vi "TC10 Update.vi"(5 "TC10 State LED ref":refnum<vi>, 7 "INTERFACE NAME ref":refnum<vi>, 8 "error in":errorcluster, 11 "XNET Session in":refnum<k21>) -> (0 "error out":errorcluster, 3 "XNET Session out":refnum<k21>)   [LabVIEW 2025, in "Automotive Ethernet Bus Monitor UI.lvlib"]
doc: "Update the TC10 session and state LED."
uses:
  Automotive Ethernet Bus Monitor UI.lvlib
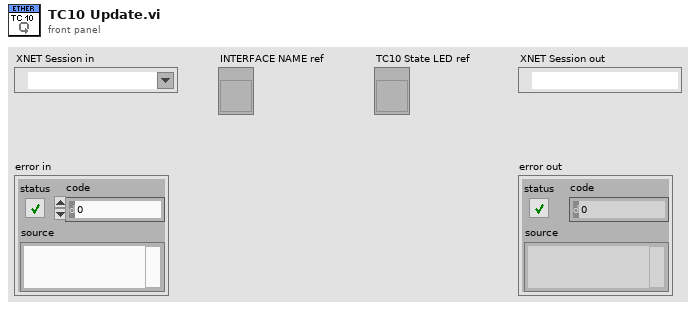
[diagram p1: front panel]
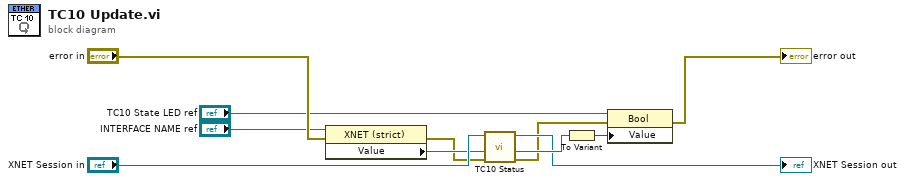
[diagram p0: block diagram]
diagram:
  n1 = property class="XNET (strict)"(reference="INTERFACE NAME ref", error in="error in") -> (error out=w3:errorcluster, "Value"=w5:refnum<k21>)  [unwired: 1 out]
  n2 = call "TC10 Status.vi"("error in (no error)"=w3, "Interface Name"=w5, "XNET Session"="XNET Session in") -> ("error out"=w4:errorcluster, "TC10 Mode"=w8:bool, "XNET Session Out"=→"XNET Session out":refnum<k21>)  [unwired: 6 in]
  n3 = To Variant(anything=w8) -> (Variant=w9:variant)
  n4 = property class="Bool"(reference="TC10 State LED ref", error in=w4, "Value"=w9) -> (error out=→"error out":errorcluster)  [unwired: 1 out]
